vi "Find Vireo Component Ids.vi"(7 "Vireo Target ID":string, 10 "error in (no error)":errorcluster, 11 "XML in":refnum<k20>) -> (2 "error out":errorcluster, 3 "XML":refnum<k20>, 5 "Vireo Component Ids":string[](array[string]))   [LabVIEW 2020, in "PicoG-Processor.lvlib" / "WebProjectWatcher.lvclass"]
uses:
  WebProjectWatcher.lvclass
  <vilib>/xml/Close Reference(Node).vi
  <vilib>/xml/NI_XML.lvlib
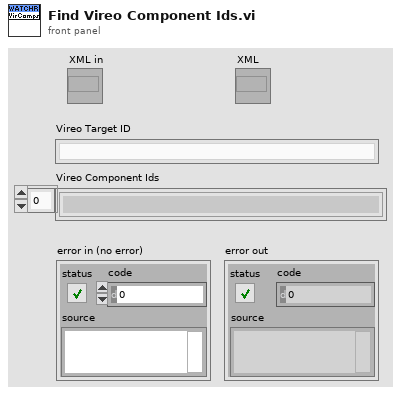
[diagram p1: front panel]
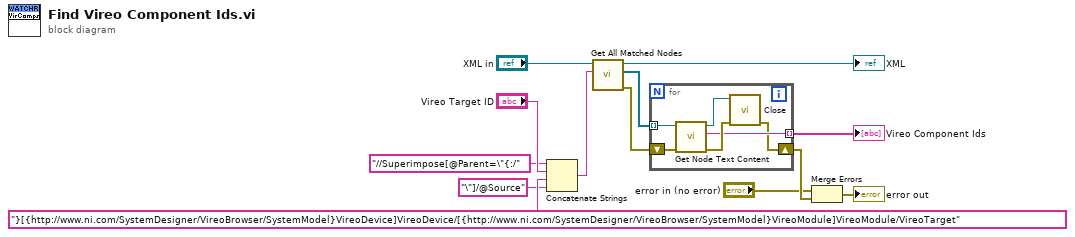
[diagram p0: block diagram]
diagram:
  n1 = Concatenate Strings("//Superimpose[@Parent=\"{:/" ("string"), "Vireo Target ID", "}[{http://www.ni.com/SystemDesigner/VireoBrowser/SystemModel}VireoDevice]VireoDevice/[{http://www.ni.com/SystemDesigner/VireoBrowser/SystemModel}VireoModule]VireoModule/VireoTarget", "\"]/@Source" ("string")) -> (w9:string)
  n2 = call <vilib>:"Get All Matched Nodes.vi"("XPath expression"=w9, "node in"="XML in") -> ("error out"=w1:errorcluster, "node result array"=w6:refnum<k20>[], "node out"=→"XML":refnum<k20>)  [unwired: 7 in]
  n3 = for {
    tunnel: w6 -> [w19] mode=indexing
    tunnel: [w16] -> w5 mode=indexing
    shift-right: [w15] -> w4
    shift-left: w1 -> [w14]
    n4 = call <vilib>:"Get Node Text Content.vi"("error in (no error)"=w14, "node in"=w19) -> ("error out"=w17:errorcluster, "node text"=w16:string, "node out"=w18:refnum<k20>)  [unwired: 7 in]
    n5 = call-poly <vilib>:"Close.vi"("error in (no error)"=w17, "node"=w18) -> ("error out"=w15:errorcluster)  [unwired: 7 in]
  }
  "Vireo Component Ids" <- w5
  n6 = Merge Errors("error in (no error)", w4) -> (→"error out":errorcluster)
